vi "Gerador de sinais - Produtor consumidor.vi"() -> ()   [LabVIEW 2019]
doc: "Use this template to build a producer/consumer design pattern with events to produce queue items. Use this design pattern instead of the User Interface Event Handler pattern for user interfaces when you want to execute code asynchronously in response to an event without slowing the user interface responsiveness."
uses:
  Data.ctl
  <vilib>/measure/NI_MABase.lvlib
panel:
  out "Forma de Onda":waveform(dbl)(graph)
  in  "Razão cíclica (%)":dbl=50.0 format="%0.2f"
  in  "Informação\nde amostragem":cluster{"Fs":dbl, "#s":dbl}={"Fs"=1000.0, "#s"=1000.0} {"Fs" format="%.2p"}
  in  "Fase":dbl format="%.2p"
  in  "Amplitude":dbl=1.0 min=0.1 step=0.1 format="%0.2p"
  in  "Frequência":dbl=10.0 format="%0.2p"
  in  "Sinal":T1(ring)
  in  "Offset":dbl format="%0.2p"
  in  "stop":bool
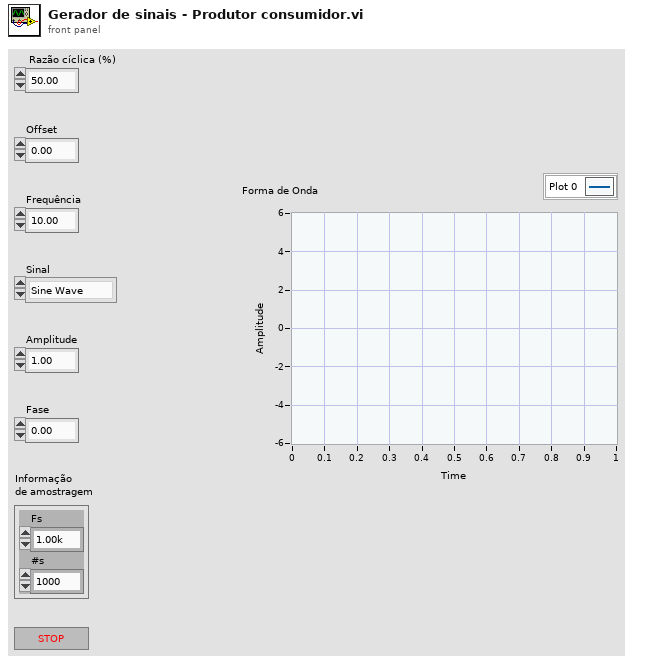
[diagram p1: front panel]
types:
  T1 = enum16{"Sine Wave", "Triangle Wave", "Square Wave", "Sawtooth Wave"}
  T2 = typedef "Data.ctl" = cluster{"Estados":enum16{"Gerar onda", "Stop"}, "Amplitude":dbl, "Informação\nde amostragem":cluster{"Fs":dbl, "#s":dbl}, "Frequência":dbl, "Offset":dbl, "Fase":dbl, "Razão cíclica (%)":dbl, "Sinal":enum16{"Sine Wave", "Triangle Wave", "Square Wave", "Sawtooth Wave"}}
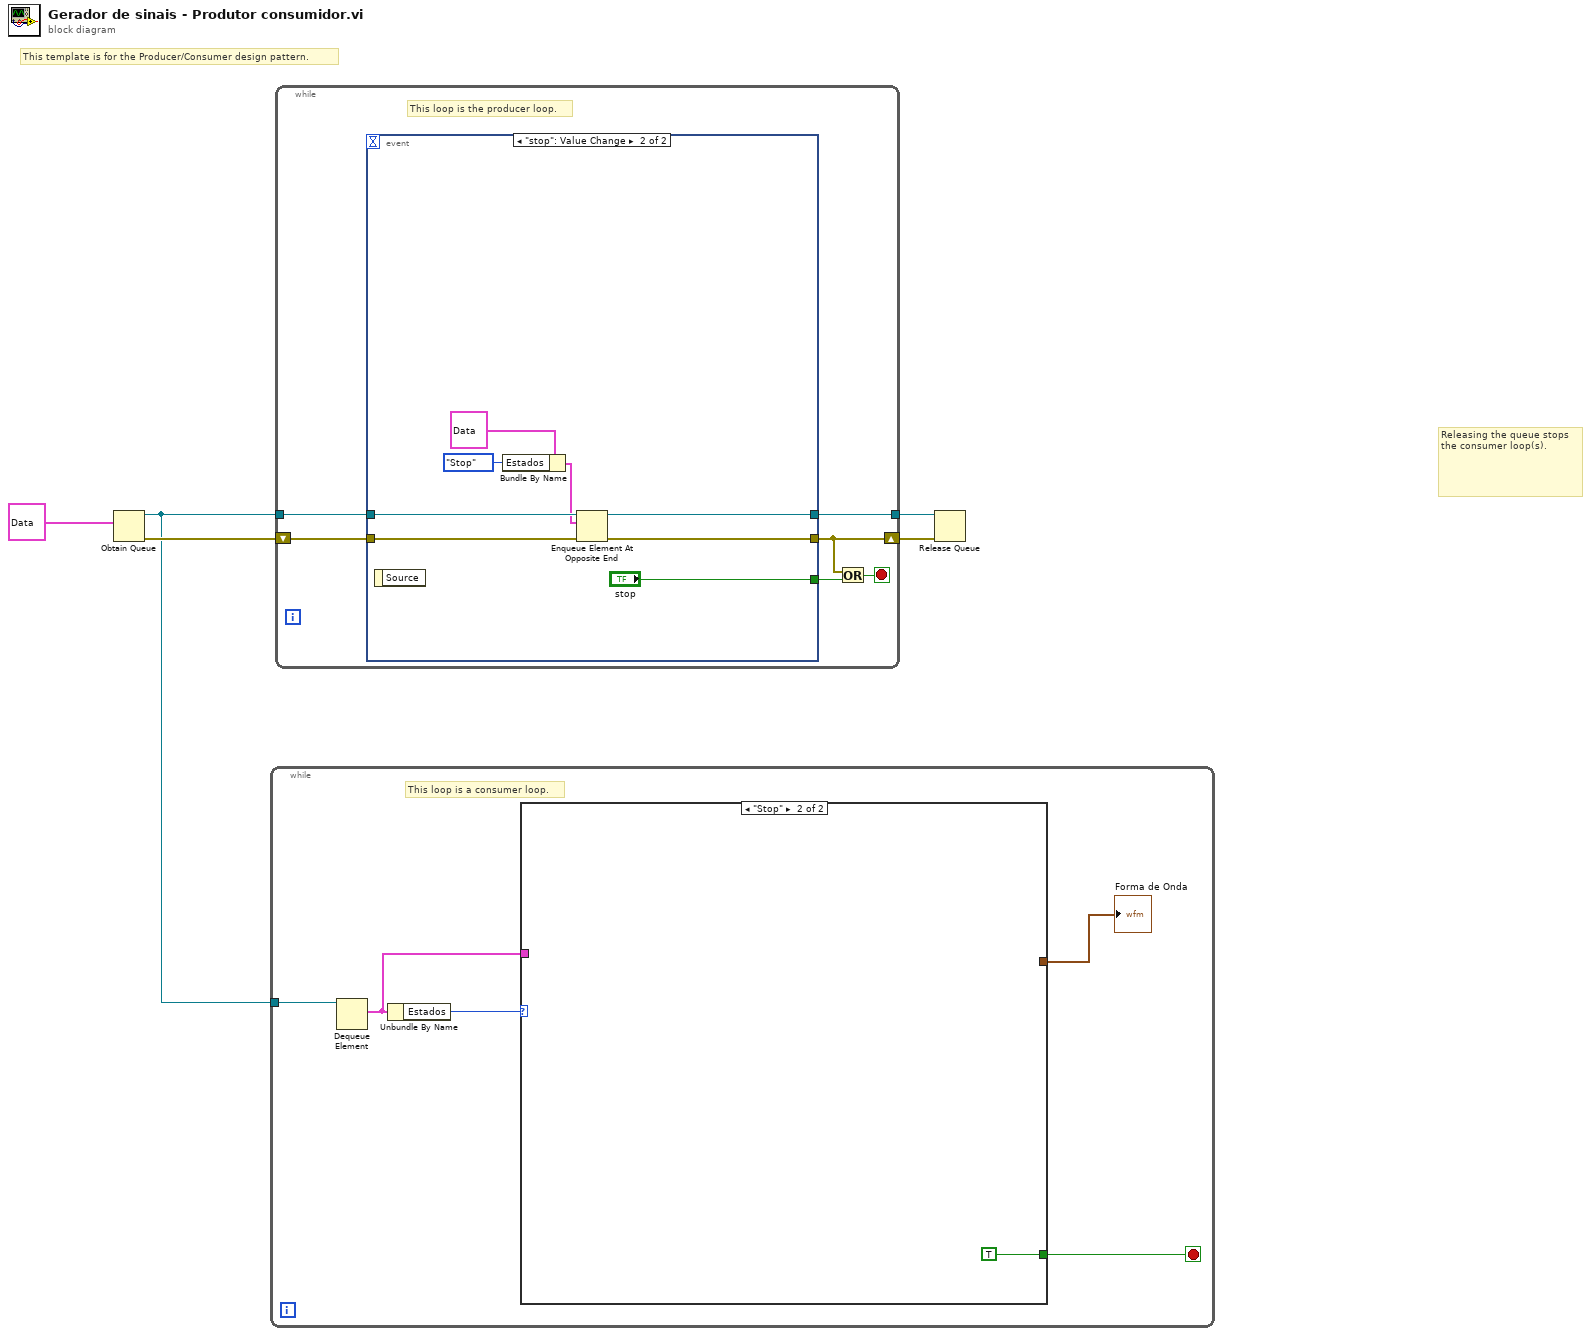
[diagram p0: block diagram]
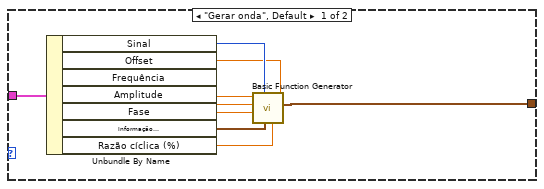
[diagram p2: hidden frame]
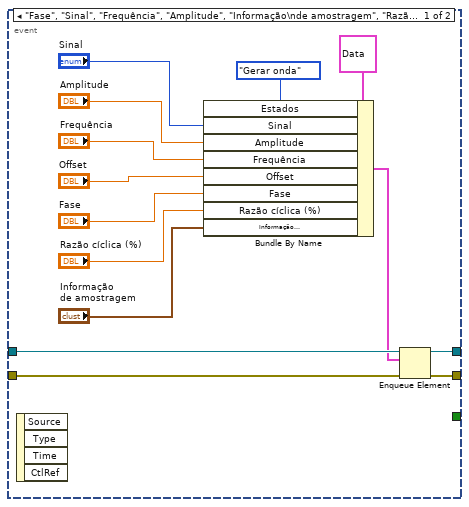
[diagram p3: hidden frame]
diagram:
  # "Releasing the queue stops the consumer loop(s)."
  # "This template is for the Producer/Consumer design pattern."
  n1 = Obtain Queue(element data type=T2 {"Estados"=enum."Gerar onda", "Amplitude"=0.0, "Informação\nde amostragem"={"Fs"=1000.0, "#s"=1000.0}, "Frequência"=0.0, "Offset"=0.0, "Fase"=0.0, "Razão cíclica (%)"=0.0, "Sinal"=enum."Sine Wave"}) -> (queue out=w2:refnum<queue>, error out=w5:errorcluster)  [unwired: 4 in, 1 out]
  n2 = while {
    tunnel: w2 -> [w10]
    stop <- w6 stop-if-true
    # "This loop is a consumer loop."
    n3 = Dequeue Element(queue=w10) -> (element=w7:T2)  [unwired: 2 in, 3 out]
    n4 = Unbundle By Name(w7) -> ("Estados"=w9:enum16{"Gerar onda", "Stop"})
    n5 = case shown="\"Stop\"" w9 {
      tunnel: w7 -> [w19 _]
      tunnel: [w11 _] -> w8
      tunnel: [_ TRUE] -> w6
      frame "Gerar onda", Default {
        n6 = Unbundle By Name(w19) -> ("Sinal"=w18:T1, "Offset"=w17:dbl, "Frequência"=w16:dbl, "Amplitude"=w15:dbl, "Fase"=w14:dbl, "Informação\nde amostragem"=w13:cluster{"Fs":dbl, "#s":dbl}, "Razão cíclica (%)"=w12:dbl)
        n7 = call <vilib>:"Basic Function Generator.vi"("offset"=w17, "square wave duty cycle (%)"=w12, "sampling info"=w13, "signal type"=w18, "phase"=w14, "amplitude"=w15, "frequency"=w16) -> ("signal out"=w11:waveform(dbl))  [unwired: 2 in, 2 out]
      }
      frame "Stop" {
      }
    }
    "Forma de Onda" <- w8
  }
  n8 = while {
    shift-right: [w22] -> w4
    shift-left: w5 -> [w25]
    tunnel: w2 -> [w26]
    tunnel: [w21] -> w1
    stop <- w23 stop-if-true
    # "This loop is the producer loop."
    n9 = event shown="[1] \"stop\": Value Change" {
      selector: _ -> [_ _]
      dyn-events: _ -> [_ _]
      timeout: _ -> [_ _]
      tunnel: w26 -> [w40 w45]
      tunnel: w25 -> [w39 w47]
      tunnel: [w38 w46] -> w22
      tunnel: [_ "stop"] -> w24
      tunnel: [w27 w44] -> w21
      event "Fase", "Sinal", "Frequência", "Amplitude", "Informação\nde amostragem", "Razão cíclica (%)", "Offset": Value Change {
        n10 = event-data() -> ()  [unwired: 1 in, 4 out]
        n11 = Bundle By Name(cluster=T2 {"Estados"=enum."Gerar onda", "Amplitude"=0.0, "Informação\nde amostragem"={"Fs"=1000.0, "#s"=1000.0}, "Frequência"=0.0, "Offset"=0.0, "Fase"=0.0, "Razão cíclica (%)"=0.0, "Sinal"=enum."Sine Wave"}, "Estados"=enum16{"Gerar onda", "Stop"}."Gerar onda", "Sinal"="Sinal", "Amplitude"="Amplitude", "Frequência"="Frequência", "Offset"="Offset", "Fase"="Fase", "Razão cíclica (%)"="Razão cíclica (%)", "Informação\nde amostragem"="Informação\nde amostragem") -> (w28:T2)
        n12 = Enqueue Element(queue=w40, element=w28, error in (no error)=w39) -> (queue out=w27:refnum<queue>, error out=w38:errorcluster)  [unwired: 1 in, 1 out]
      }
      event "stop": Value Change {
        n13 = event-data() -> ()  [unwired: 1 in, 1 out]
        n14 = Bundle By Name(cluster=T2 {"Estados"=enum."Gerar onda", "Amplitude"=0.0, "Informação\nde amostragem"={"Fs"=1000.0, "#s"=1000.0}, "Frequência"=0.0, "Offset"=0.0, "Fase"=0.0, "Razão cíclica (%)"=0.0, "Sinal"=enum."Sine Wave"}, "Estados"=enum16{"Gerar onda", "Stop"}."Stop") -> (w42:T2)
        n15 = Enqueue Element At Opposite End(queue=w45, element=w42, error in (no error)=w47) -> (queue out=w44:refnum<queue>, error out=w46:errorcluster)  [unwired: 1 in, 1 out]
      }
    }
    n16 = Or(x=w22, y=w24) -> (x .or. y?=w23:bool)
  }
  n17 = Release Queue(queue=w1, error in (no error)=w4) -> ()  [unwired: 1 in, 3 out]
